vi "Generate Unified Msg Set.vi"(11 "TEMPLATE Actor in":refnum<class "TEMPLATE Actor.lvclass">) -> (2 "Unified Msg Set":T1)   [LabVIEW 2020, in "_Template.lvlib" / "Templates.lvlib" / "TEMPLATE Actor.lvlib" / "TEMPLATE Actor.lvclass"]
uses:
  TEMPLATE Actor.lvclass
  jettl/jettl/Actor/Actor/Actor.lvclass
  jettl/jettl/Msg/Msg.lvclass
  jettl/jettl/Actor/Msg Set.ctl
  jettl/jettl/Actor/Actor.lvlib
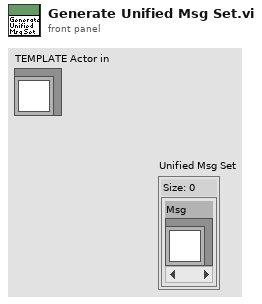
[diagram p1: front panel]
types:
  T1 = typedef "jettl.lvlib/Actor.lvlib/Msg Set.ctl" = set{refnum<class "Msg.lvclass">}
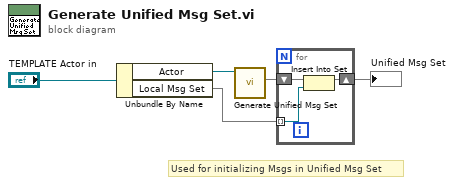
[diagram p0: block diagram]
diagram:
  # "Used for initializing Msgs in Unified Msg Set"
  n1 = Unbundle By Name("TEMPLATE Actor in") -> ("Actor"=w5:refnum<class "Actor.lvclass">, "Local Msg Set"=w1:T1)
  n2 = call-dynamic "Generate Unified Msg Set.vi"("Get Actor in"=w5) -> ("Unified Msg Set"=w4:T1)  [unwired: 10 in]
  n3 = for {
    tunnel: w1 -> [w7] mode=indexing
    shift-right: [w6] -> w3
    shift-left: w4 -> [w8]
    n4 = Insert Into Set(10:w7, 11:w8) -> (3:w6:T1)  [unwired: 1 out]
  }
  "Unified Msg Set" <- w3
